vi "Main Window.vi"() -> ()   [LabVIEW 2015]
uses:
  Control Button/Exit.ctl
  Control Button/login.ctl
  Control Button/Logout.ctl
  Control Button/setting.ctl
  Control Button/report.ctl
  Control Button/Manual.ctl
  Control Button/Start.ctl
  Enqueue/Main window Seq/Test selection_1.ctl
  Enqueue/Main window Seq/Test seq_1.ctl
  Galobal variable_TI.vi
  Project Setup/Globle Variable/GR_Servo.vi
panel:
  out "Boolean 3":bool
  out "error out 2":errorcluster
  out "Boolean 2":bool
  out "Error 2":bool
  out "Error":bool
  out "User Name":string
  out "error out":errorcluster
  out "x = y?":bool
  out "Company Name":string
  in  "Sign In":T1
  out "Boolean":bool
  in  "Dashbord":T6
  in  "Login Window":T8 {"User Name" items=["admin", "mmum", "a", "AJAY Kumar", "", "", "", "", "", "", "", "", "", "", "", "", "", "", "", "", "", "", "", "", "", "", "", "", "", "", "", ""]}
  in  "Exit":T9
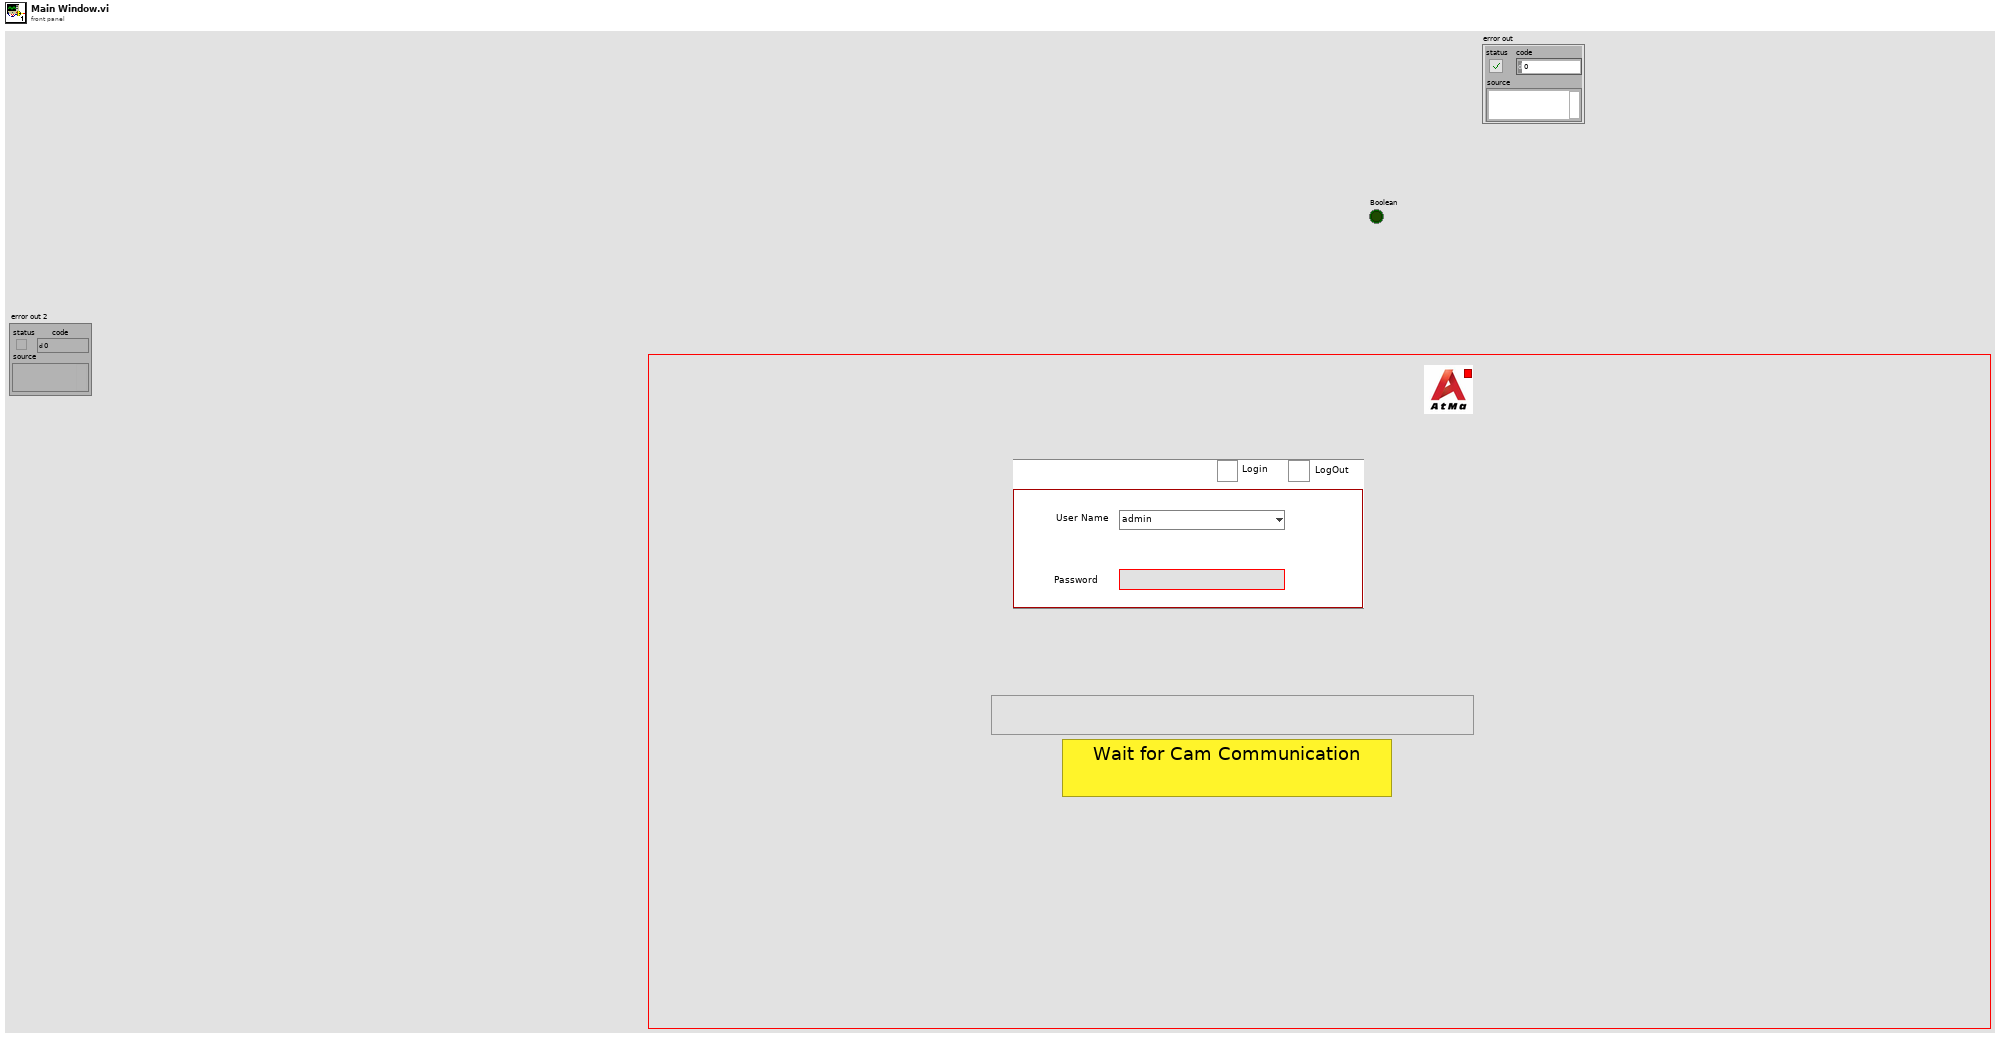
[diagram p1: front panel]
types:
  T1 = typedef "login.ctl" = bool
  T2 = typedef "setting.ctl" = bool
  T3 = typedef "report.ctl" = bool
  T4 = typedef "Manual.ctl" = bool
  T5 = typedef "Start.ctl" = bool
  T6 = cluster{"Setting":T2, "Report":T3, "Manaul":T4, "Start":T5}
  T7 = typedef "Logout.ctl" = bool
  T8 = cluster{"User Name":u16, "Password":string, "Sign In":T1, "Log Out":T7}
  T9 = typedef "Exit.ctl" = bool
  T10 = typedef "Test selection_1.ctl" = enum16{"Init", "Enqueue ", "Enqueue N", "Enqueue in stack", "Enqueue in stack N", "Dequeue", "Dequeue N", "Flush", "Release Queue"}
  T11 = typedef "Test seq_1.ctl" = enum16{"Poll Event", "Login", "Logout", "Confi", "Manual", "Report", "Testing", "Exit"}
  T12 = cluster{"XInput":dbl[], "Y New Value":dbl[], "Avg point":i16}[]
  T13 = cluster{"Slop":dbl[], "Intercept":dbl[], "Average ":i16[]}
  T14 = cluster{"UserName":string[], "Password":string[], "Usertype":string[], "Analog Min":string[], "Analog Max":string[], "DigitalInput Port":string[], "Digital Output Port":string[], "ANalog Port":string[], "IOList":cluster{"DI List_280":string[], "D0List _280":string[], "AI List_280":string[]}}
  T15 = cluster{"DI List_280":string[], "D0List _280":string[], "AI List_280":string[]}
  T16 = cluster{"DigitalInput Port[0]":string, "DigitalInput Port[1]":string, "DigitalInput Port[2]":string, "DigitalInput Port[3]":string, "DigitalInput Port[4]":string, "DigitalInput Port[5]":string, "DigitalInput Port[6]":string, "DigitalInput Port[7]":string, "DigitalInput Port[8]":string, "DigitalInput Port[9]":string, "DigitalInput Port[10]":string, "DigitalInput Port[11]":string, "DigitalInput Port[12]":string, "DigitalInput Port[13]":string, "DigitalInput Port[14]":string, "DigitalInput Port[15]":string}
  T17 = cluster{"Digital Output Port[0]":string, "Digital Output Port[1]":string, "Digital Output Port[2]":string, "Digital Output Port[3]":string, "Digital Output Port[4]":string, "Digital Output Port[5]":string, "Digital Output Port[6]":string, "Digital Output Port[7]":string, "Digital Output Port[8]":string, "Digital Output Port[9]":string, "Digital Output Port[10]":string, "Digital Output Port[11]":string, "Digital Output Port[12]":string, "Digital Output Port[13]":string, "Digital Output Port[14]":string, "Digital Output Port[15]":string, "Digital Output Port[16]":string, "Digital Output Port[17]":string, "Digital Output Port[18]":string, "Digital Output Port[19]":string, "Digital Output Port[20]":string, "Digital Output Port[21]":string, "Digital Output Port[22]":string, "Digital Output Port[23]":string, "Digital Output Port[24]":string, "Digital Output Port[25]":string, "Digital Output Port[26]":string, "Digital Output Port[27]":string, "Digital Output Port[28]":string, "Digital Output Port[29]":string}
  T18 = cluster{"ANalog Port[0]":string, "ANalog Port[1]":string, "ANalog Port[2]":string, "ANalog Port[3]":string, "ANalog Port[4]":string, "ANalog Port[5]":string, "ANalog Port[6]":string, "ANalog Port[7]":string, "ANalog Port[8]":string, "ANalog Port[9]":string, "ANalog Port[10]":string, "ANalog Port[11]":string, "ANalog Port[12]":string, "ANalog Port[13]":string, "ANalog Port[14]":string, "ANalog Port[15]":string, "ANalog Port[16]":string, "ANalog Port[17]":string, "ANalog Port[18]":string, "ANalog Port[19]":string, "ANalog Port[20]":string, "ANalog Port[21]":string, "ANalog Port[22]":string, "ANalog Port[23]":string, "ANalog Port[24]":string, "ANalog Port[25]":string, "ANalog Port[26]":string, "ANalog Port[27]":string, "ANalog Port[28]":string, "ANalog Port[29]":string, "ANalog Port[30]":string, "ANalog Port[31]":string}
  T19 = enum32{"Invalid", "Standard", "Closed", "Hidden", "Minimized", "Maximized"}
  T20 = enum8{"Enabled", "Disabled", "Disabled and Grayed Out"}
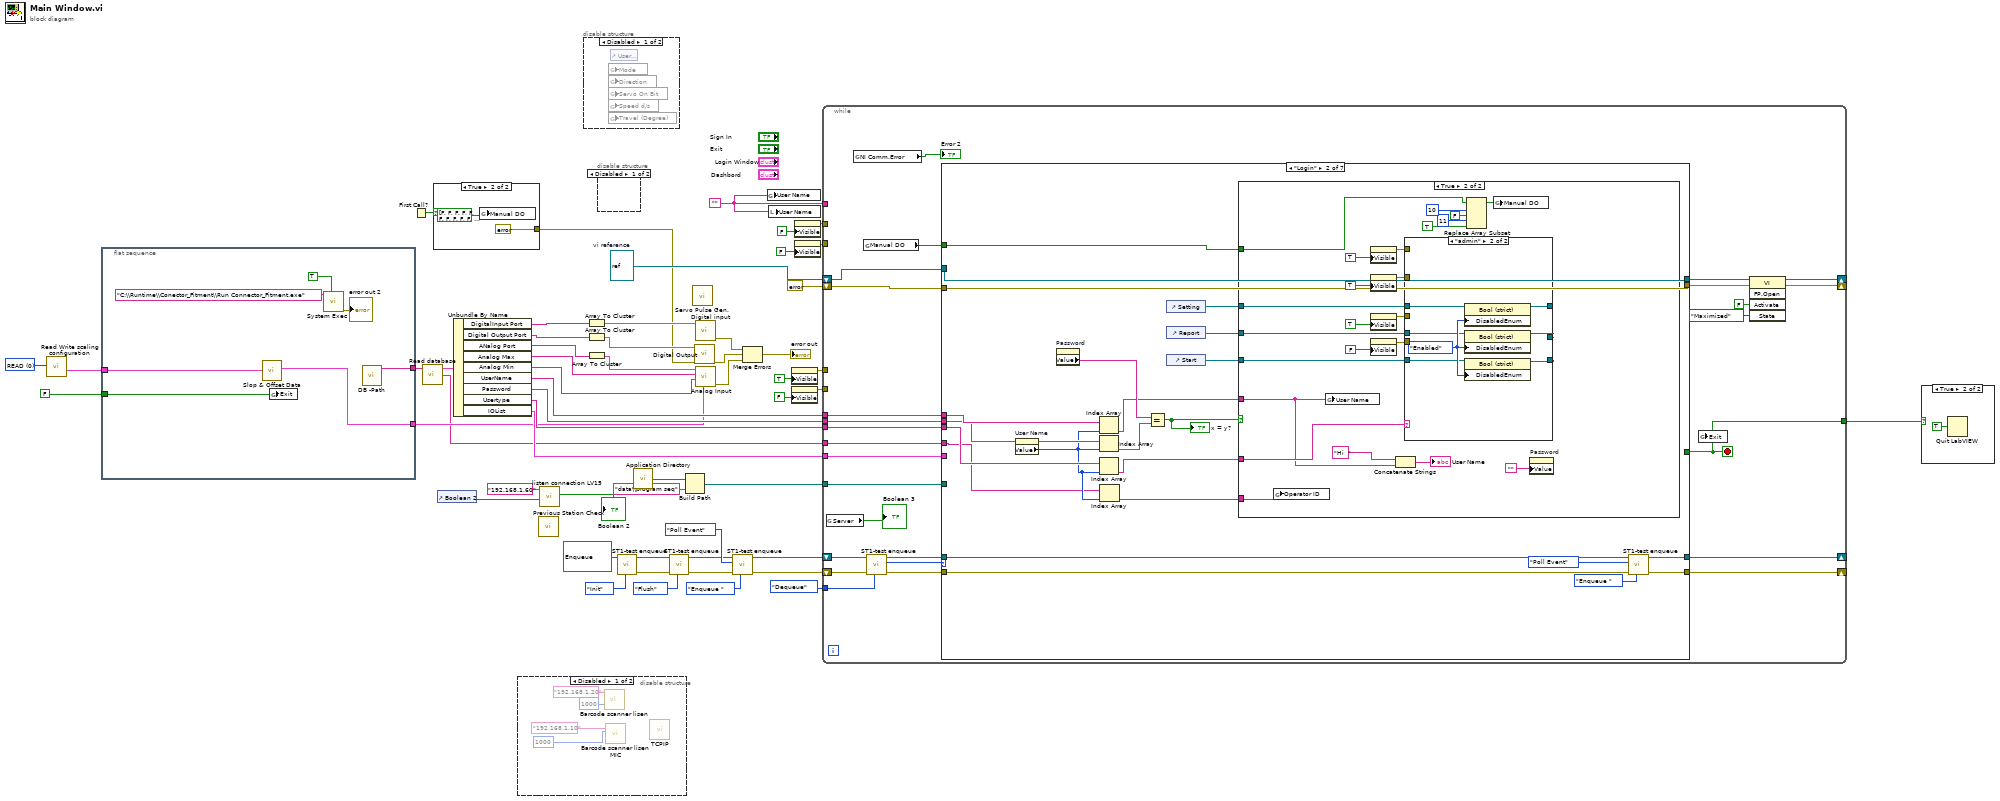
[diagram p0: block diagram]
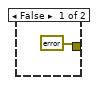
[diagram p5: hidden frame]
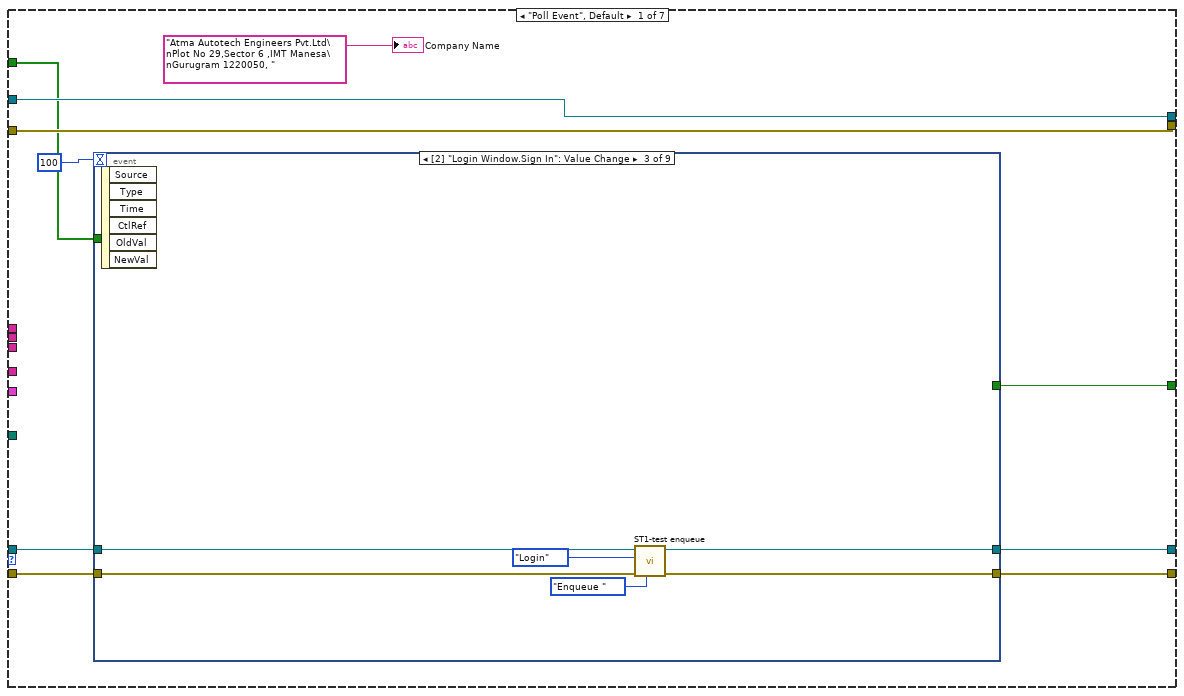
[diagram p7: hidden frame]
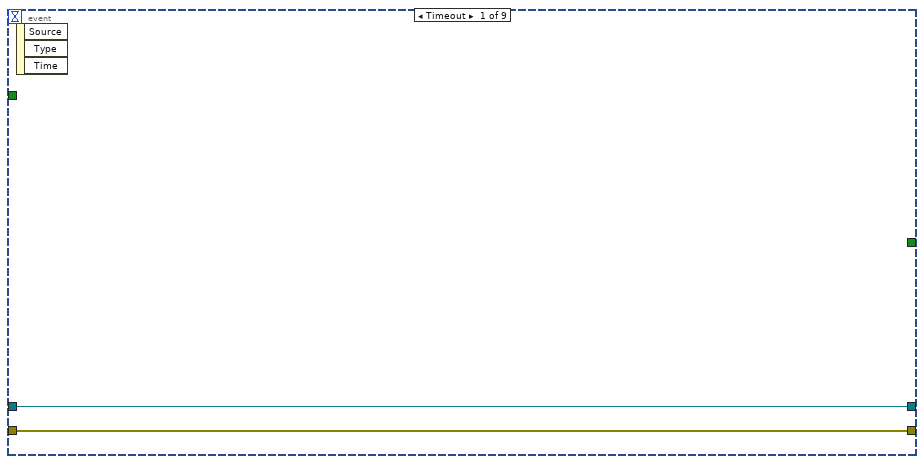
[diagram p8: hidden frame]
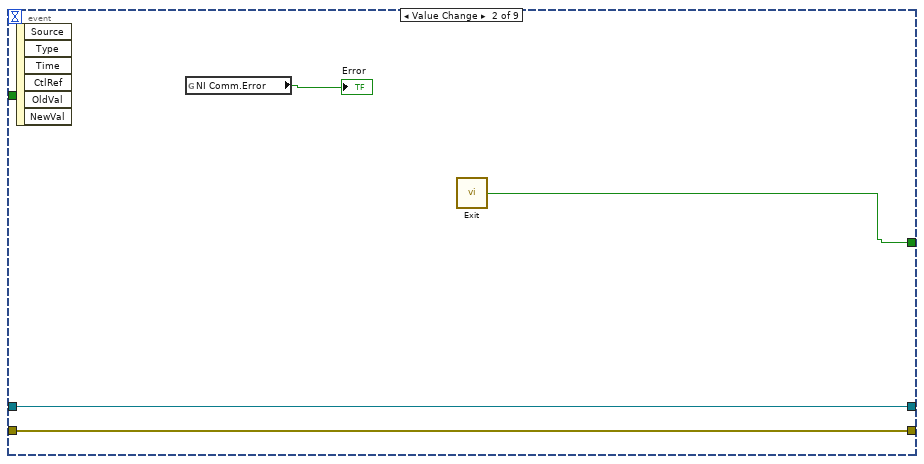
[diagram p9: hidden frame]
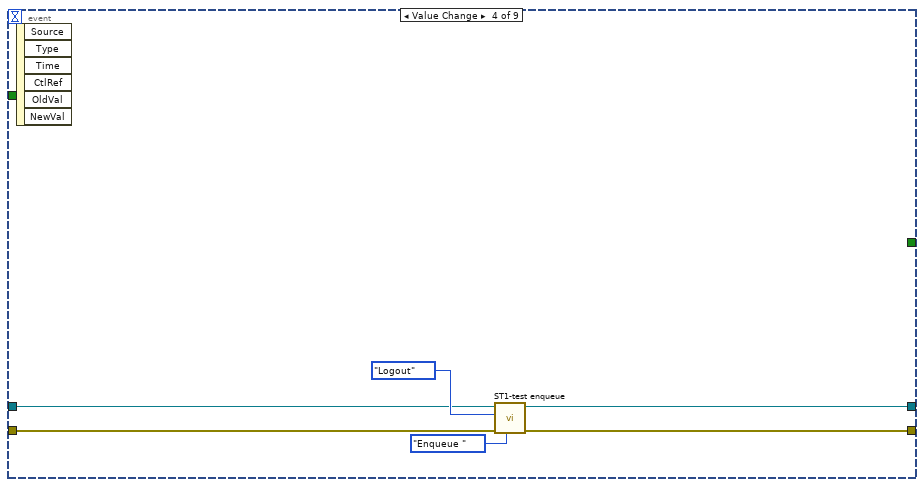
[diagram p10: hidden frame]
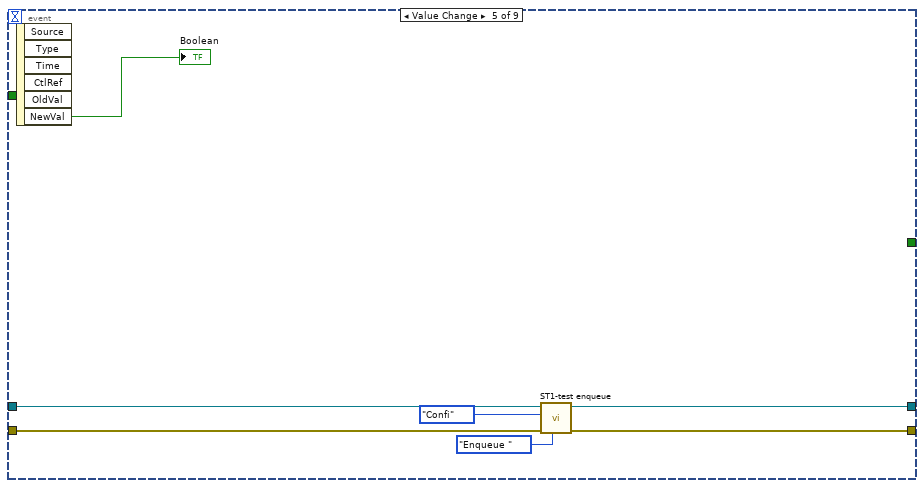
[diagram p11: hidden frame]
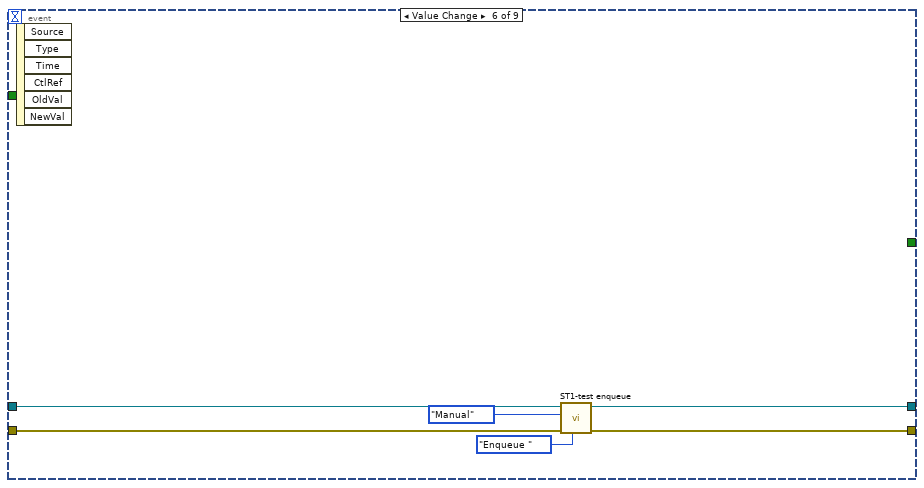
[diagram p12: hidden frame]
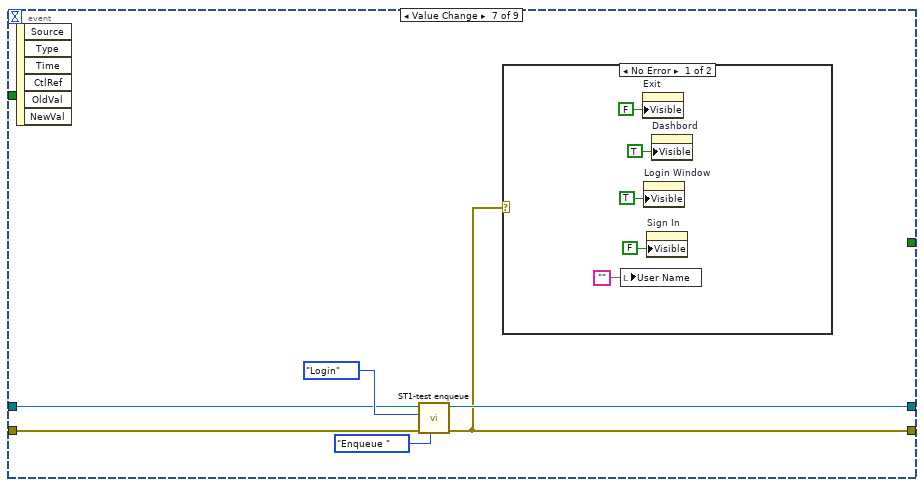
[diagram p13: hidden frame]
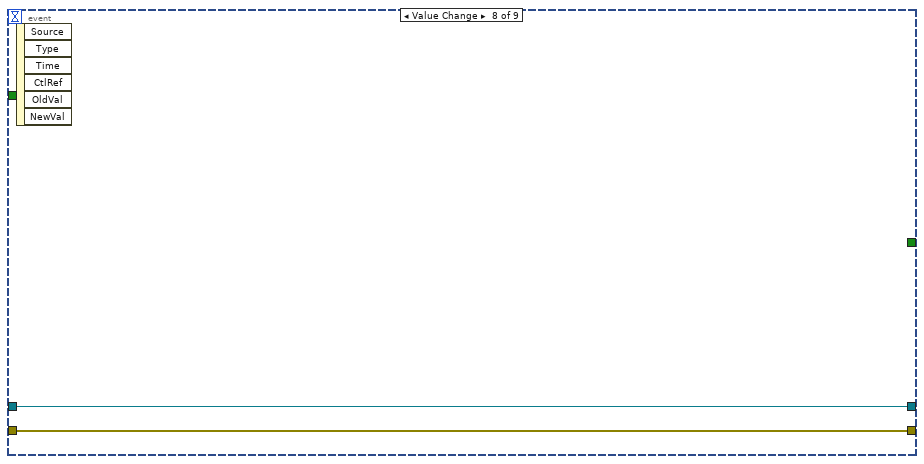
[diagram p15: hidden frame]
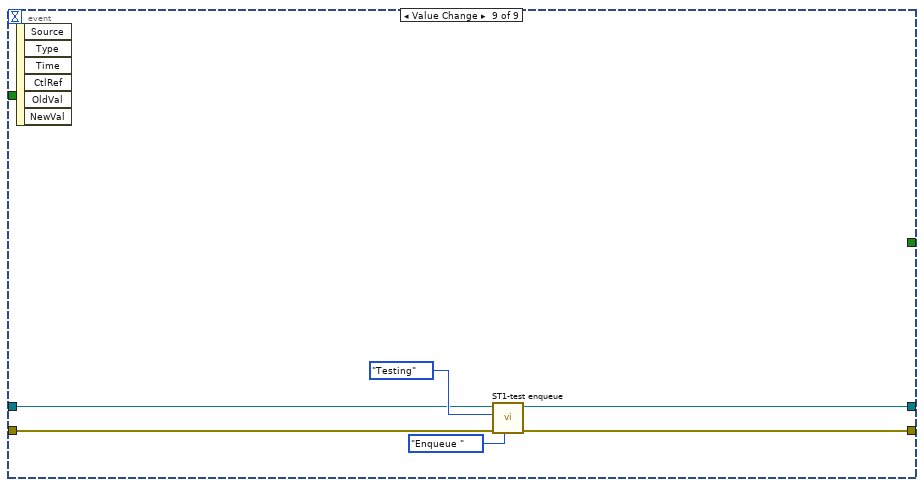
[diagram p16: hidden frame]
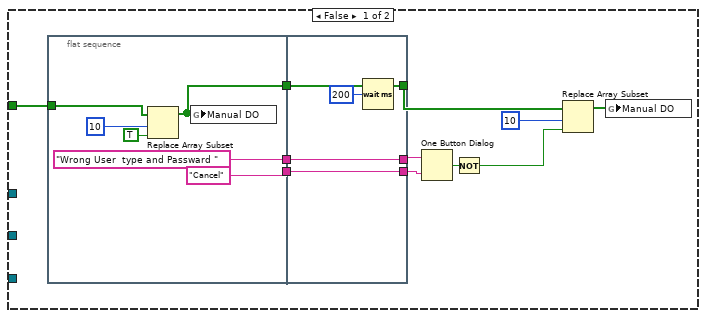
[diagram p17: hidden frame]
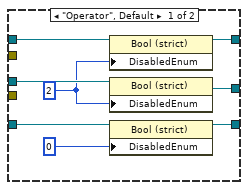
[diagram p18: hidden frame]
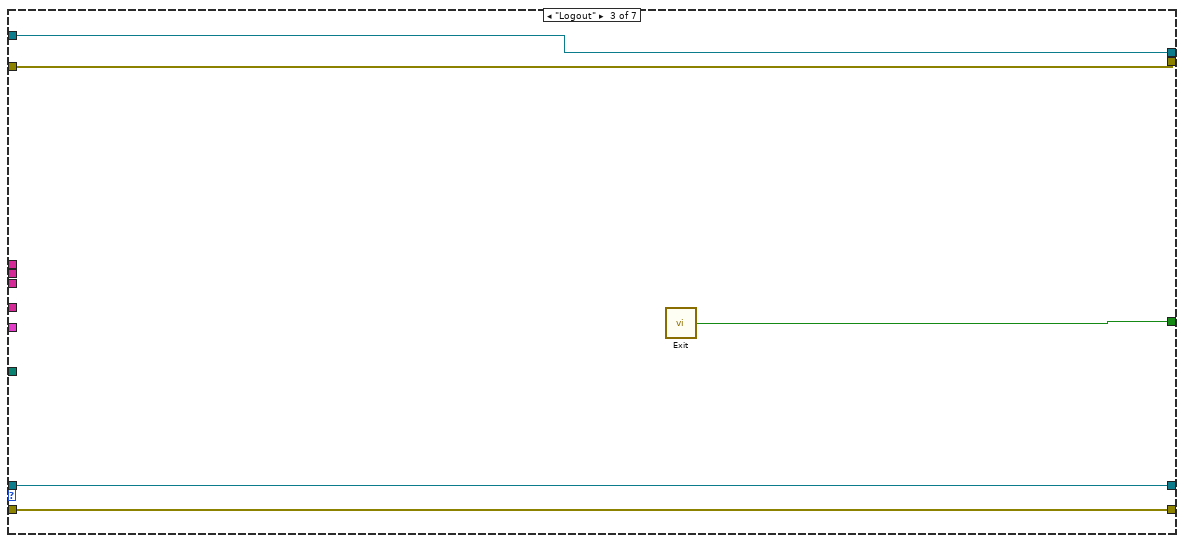
[diagram p19: hidden frame]
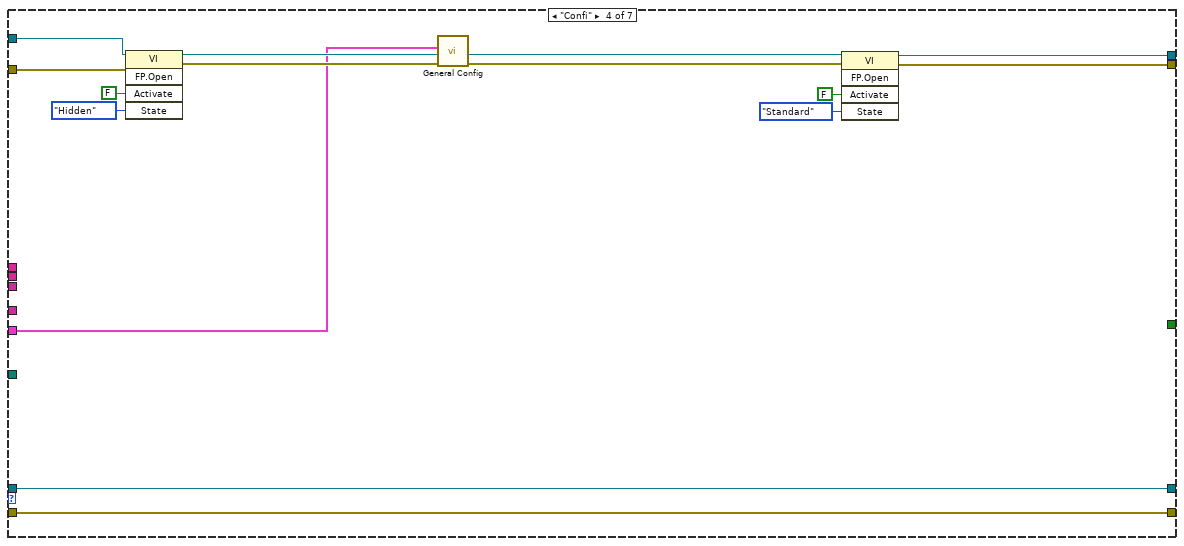
[diagram p20: hidden frame]
diagram:
  w18 = u16 0 items=["READ", "WRITE"] ("Read/Write")
  w33 = ""
  w43 = refnum<vi> refnum  # vi reference
  w44 = refnum<queue> refnum items=["Poll Event", "Login", "Logout", "Confi", "Manual", "Report", "Testing", "Exit"] ("queue in")
  n1 = call "Read Write scaling configuration.vi"("Read/Write"=w18) -> ("Output"=w17:T12)  [unwired: 4 in, 2 out]
  n2 = flat-sequence {
    tunnel: [w62] -> w32
    tunnel: w17 -> [w61]
    tunnel: [w60] -> w16
    tunnel: FALSE ("Exit") -> [w59]
    frame #0 {
      n3 = call "Slop & Offset Data.vi"("Input"=w61) -> ("Cluster"=w60:T13)  [unwired: 10 in]
      n4 = global write "Galobal variable_TI.vi" "Exit"(w59) -> ()
      n5 = call <vilib>:"System Exec.vi"("wait until completion? (T)"=TRUE, "command line"="C:\\Runtime\\Conector_Fitment\\Run Connector_Fitment.exe") -> ("error out"=→"error out 2":errorcluster)  [unwired: 6 in, 3 out]
      n6 = call "DB -Path.vi"() -> ("String"=w62:string)  [unwired: 11 in]
    }
  }
  n7 = First Call?() -> (First Call?: T/F=w7:bool)
  n8 = call "Read database.vi"("String"=w32) -> ("Operator Id"=w1:string[], "DB Data"=w31:T14)  [unwired: 2 in, 1 out]
  n9 = case shown="True" w7 {
    tunnel: [errorcluster {"status"=FALSE, "code"=0, "source"=""} ("error constant") errorcluster {"status"=FALSE, "code"=0, "source"=""} ("error constant")] -> w6
    frame False {
    }
    frame True {
      n10 = global write "Galobal variable_TI.vi" "Manual DO"(bool[] [FALSE, FALSE, FALSE, FALSE, FALSE, FALSE, FALSE, FALSE, FALSE, FALSE, FALSE, FALSE, FALSE, FALSE, FALSE, FALSE, FALSE, FALSE, FALSE, FALSE, FALSE, FALSE, FALSE, FALSE, FALSE, FALSE, FALSE, FALSE, FALSE, FALSE] ("Manual DO")) -> ()
    }
  }
  n11 = control-ref of="Boolean 2"() -> (w3:refnum<vi>)
  n12 = Unbundle By Name(w31) -> ("DigitalInput Port"=w30:string[], "Digital Output Port"=w28:string[], "ANalog Port"=w26:string[], "Analog Max"=w24:string[], "Analog Min"=w23:string[], "UserName"=w22:string[], "Password"=w21:string[], "Usertype"=w20:string[], "IOList"=w19:T15)
  n13 = disable-structure shown="Disabled" {
    frame Disabled {
      n14 = call "Barcode scanner lisen.vi"("port"=u16 1000, "service name"="192.168.1.20") -> ()  [unwired: 7 in, 3 out]
      n15 = call "Barcode scanner lisen MIC.vi"("port"=u16 1000, "service name"="192.168.1.10") -> ()  [unwired: 7 in, 3 out]
      n16 = call "TCPIP.vi"() -> ()  [unwired: 12 in]
    }
    frame Enabled {
    }
  }
  n17 = call "Previous Station Check.vi"() -> ()  [unwired: 12 in]
  n18 = call "listen connection LV15.vi"("Bool Refnum"=w3, "service name"="192.168.1.60") -> ("Boolean 3"=→"Boolean 2":bool)  [unwired: 7 in, 1 out]
  n19 = disable-structure shown="Disabled" {
    frame Disabled {
      n20 = global read "GR_Servo.vi" "Mode"() -> ()  [unwired: 1 in]
      n21 = global read "GR_Servo.vi" "Direction"() -> ()  [unwired: 1 in]
      n22 = global read "GR_Servo.vi" "Servo On Bit"() -> ()  [unwired: 1 in]
      n23 = global read "GR_Servo.vi" "Speed d/s"() -> ()  [unwired: 1 in]
      n24 = global read "GR_Servo.vi" "Travel (Degree)"() -> ()  [unwired: 1 in]
      n25 = control-ref of="User Name"() -> ()  [unwired: 1 out]
    }
    frame Enabled {
    }
  }
  n26 = Array To Cluster(array=w30) -> (cluster=w29:T16)
  n27 = Array To Cluster(array=w28) -> (cluster=w27:T17)
  n28 = Array To Cluster(array=w26) -> (cluster=w25:T18)
  n29 = disable-structure shown="Disabled" {
    frame Disabled {
    }
    frame Enabled {
    }
  }
  n30 = call "ST1-test enqueue.vi"("Enum Selection"=Test_selection_1."Init", "queue in"=w44) -> ("error out"=w53:errorcluster, "queue Out"=w49:refnum<queue>)  [unwired: 6 in, 1 out]
  n31 = call <vilib>:"Application Directory.vi"() -> ("Application Directory"=w10:path)
  n32 = call "ST1-test enqueue.vi"("Enum Selection"=Test_selection_1."Flush", "Error In"=w53, "queue in"=w49) -> ("error out"=w51:errorcluster, "queue Out"=w48:refnum<queue>)  [unwired: 5 in, 1 out]
  n33 = Build Path(base path=w10, name or relative path="data\\program seq") -> (appended path=w8:path)
  n34 = call "Servo Pulse Gen..vi"() -> ()  [unwired: 12 in]
  n35 = call "Digital Output.vi"("error in"=w6, "DAQmx OutPut Setting"=w27) -> ("error out"=w14:errorcluster)  [unwired: 8 in, 1 out]
  n36 = call "Digital input.vi"("DAQmx InPut Setting"=w29) -> ("error out"=w12:errorcluster)  [unwired: 9 in, 1 out]
  n37 = call "Analog Input.vi"("clai. Parmeter"=w16, "Min Value"=w23, "Max Value"=w24, "DAQmx Analog Input Setting"=w25) -> ("error out"=w13:errorcluster)  [unwired: 6 in, 1 out]
  n38 = call "ST1-test enqueue.vi"("Enum Selection"=Test_selection_1."Enqueue ", "Error In"=w51, "Enqueue"=Test_seq_1."Poll Event", "queue in"=w48) -> ("error out"=w46:errorcluster, "queue Out"=w47:refnum<queue>)  [unwired: 4 in, 1 out]
  n39 = Merge Errors(w12, w14, w13) -> (→"error out":errorcluster)
  n40 = global write "Galobal variable_TI.vi" "User Name"(w33) -> ()
  n41 = local write "User Name"(w33) -> ()
  n42 = property on="Login Window" class="Clust (strict)"("Visible"=TRUE) -> (error out=w38:errorcluster)  [unwired: 2 in, 1 out]
  n43 = property on="Sign In" class="Bool (strict)"("Visible"=FALSE) -> (error out=w37:errorcluster)  [unwired: 2 in, 1 out]
  n44 = property on="Exit" class="Bool (strict)"("Visible"=FALSE) -> (error out=w35:errorcluster)  [unwired: 2 in, 1 out]
  n45 = property on="Dashbord" class="Clust (strict)"("Visible"=FALSE) -> (error out=w40:errorcluster)  [unwired: 2 in, 1 out]
  n46 = while {
    shift-right: [w89] -> _
    shift-left: w47 -> [w95]
    shift-right: [w88] -> _
    shift-left: w46 -> [w94]
    tunnel: Test_selection_1."Dequeue" ("Enum Selection") -> [w93]
    shift-right: [w80] -> _
    shift-left: errorcluster {"status"=FALSE, "code"=0, "source"=""} ("error out") -> [w86]
    shift-right: [w81] -> _
    shift-left: w43 -> [w87]
    tunnel: w40 -> [_]
    tunnel: w38 -> [_]
    tunnel: w37 -> [_]
    tunnel: w35 -> [_]
    tunnel: w33 -> [_]
    tunnel: w22 -> [w79]
    tunnel: w21 -> [w78]
    tunnel: w20 -> [w77]
    tunnel: w19 -> [w76]
    tunnel: w8 -> [w75]
    tunnel: [w73] -> w5
    tunnel: w1 -> [w70]
    stop <- w73 stop-if-true
    n47 = global read "Galobal variable_TI.vi" "Server"() -> (→"Boolean 3":bool)
    n48 = global read "Galobal variable_TI.vi" "NI Comm.Error"() -> (→"Error 2":bool)
    n49 = global read "Galobal variable_TI.vi" "Manual DO"() -> (w74:bool[])
    n50 = call "ST1-test enqueue.vi"("Enum Selection"=w93, "Error In"=w94, "queue in"=w95) -> ("error out"=w90:errorcluster, "D-enqueue"=w92:T11, "queue Out"=w91:refnum<queue>)  [unwired: 5 in]
    n51 = case shown="\"Login\"" w92 {
      tunnel: [w103 _ w238 _ _ _ _] -> w73
      tunnel: w91 -> [w104 w160 w242 w256 w264 w273 w290]
      tunnel: w90 -> [w105 w159 w241 w255 w263 w272 w289]
      tunnel: [w102 w163 w242 w256 w264 w273 w290] -> w89
      tunnel: [w101 w162 w241 w255 w263 w272 w289] -> w88
      tunnel: [w100 w172 w240 w250 w259 w271 w276] -> w83
      tunnel: [w99 w171 w239 w249 w260 w270 w274] -> w82
      tunnel: w87 -> [w100 w172 w240 w248 w261 w271 w282]
      tunnel: w86 -> [w99 w171 w239 w247 w262 w270 w285]
      tunnel: w79 -> [_ w169 _ _ _ _ _]
      tunnel: w78 -> [_ w168 _ _ _ _ _]
      tunnel: w77 -> [_ w167 _ _ _ _ _]
      tunnel: w76 -> [_ _ _ w243 w258 _ w288]
      tunnel: w75 -> [_ _ _ _ _ _ w280]
      tunnel: w74 -> [w96 w161 _ _ _ _ _]
      tunnel: w70 -> [_ w157 _ _ _ _ _]
      frame "Poll Event", Default {
        n52 = event shown="[2] \"Login Window.Sign In\": Value Change" {
          selector: _ -> [_ _ _ _ _ _ _ _ _]
          dyn-events: _ -> [_ _ _ _ _ _ _ _ _]
          timeout: 100 -> [_ _ _ _ _ _ _ _ _]
          tunnel: [_ w109 _ _ _ _ _ _ _] -> w103
          tunnel: w105 -> [w106 w110 w115 w118 w126 w134 w140 w148 w152]
          tunnel: w104 -> [w107 w111 w116 w119 w127 w132 w139 w149 w153]
          tunnel: [w107 w111 w114 w121 w125 w131 w138 w149 w151] -> w102
          tunnel: [w106 w110 w113 w120 w124 w133 w137 w148 w150] -> w101
          tunnel: w96 -> [_ _ _ _ _ _ _ _ _]
          event Timeout {
            n53 = event-data() -> ()  [unwired: 1 in, 3 out]
          }
          event Value Change {
            n54 = event-data() -> ()  [unwired: 1 in, 6 out]
            n55 = global read "Galobal variable_TI.vi" "NI Comm.Error"() -> (→"Error":bool)
            n56 = call "Exit.vi"() -> ("Exit"=w109:bool)  [unwired: 1 in]
          }
          event Value Change {
            n57 = event-data() -> ()  [unwired: 1 in, 6 out]
            n58 = call "ST1-test enqueue.vi"("Enum Selection"=Test_selection_1."Enqueue ", "Error In"=w115, "Enqueue"=Test_seq_1."Login", "queue in"=w116) -> ("error out"=w113:errorcluster, "queue Out"=w114:refnum<queue>)  [unwired: 4 in, 1 out]
          }
          event Value Change {
            n59 = event-data() -> ()  [unwired: 1 in, 6 out]
            n60 = call "ST1-test enqueue.vi"("Enum Selection"=Test_selection_1."Enqueue ", "Error In"=w118, "Enqueue"=Test_seq_1."Logout", "queue in"=w119) -> ("error out"=w120:errorcluster, "queue Out"=w121:refnum<queue>)  [unwired: 4 in, 1 out]
          }
          event Value Change {
            n61 = event-data() -> ("NewVal"=→"Boolean":T2)  [unwired: 1 in, 5 out]
            n62 = call "ST1-test enqueue.vi"("Enum Selection"=Test_selection_1."Enqueue ", "Error In"=w126, "Enqueue"=Test_seq_1."Confi", "queue in"=w127) -> ("error out"=w124:errorcluster, "queue Out"=w125:refnum<queue>)  [unwired: 4 in, 1 out]
          }
          event Value Change {
            n63 = event-data() -> ()  [unwired: 1 in, 6 out]
            n64 = call "ST1-test enqueue.vi"("Enum Selection"=Test_selection_1."Enqueue ", "Error In"=w134, "Enqueue"=Test_seq_1."Manual", "queue in"=w132) -> ("error out"=w133:errorcluster, "queue Out"=w131:refnum<queue>)  [unwired: 4 in, 1 out]
          }
          event Value Change {
            n65 = event-data() -> ()  [unwired: 1 in, 6 out]
            n66 = call "ST1-test enqueue.vi"("Enum Selection"=Test_selection_1."Enqueue ", "Error In"=w140, "Enqueue"=Test_seq_1."Login", "queue in"=w139) -> ("error out"=w137:errorcluster, "queue Out"=w138:refnum<queue>)  [unwired: 4 in, 1 out]
            n67 = case shown="No Error" w137 {
              frame No Error {
                n68 = local write "User Name"("") -> ()
                n69 = property on="Exit" class="Bool (strict)"("Visible"=FALSE) -> ()  [unwired: 2 in, 2 out]
                n70 = property on="Login Window" class="Clust (strict)"("Visible"=TRUE) -> ()  [unwired: 2 in, 2 out]
                n71 = property on="Sign In" class="Bool (strict)"("Visible"=FALSE) -> ()  [unwired: 2 in, 2 out]
                n72 = property on="Dashbord" class="Clust (strict)"("Visible"=TRUE) -> ()  [unwired: 2 in, 2 out]
              }
              frame Error {
              }
            }
          }
          event Value Change {
            n73 = event-data() -> ()  [unwired: 1 in, 6 out]
          }
          event Value Change {
            n74 = event-data() -> ()  [unwired: 1 in, 6 out]
            n75 = call "ST1-test enqueue.vi"("Enum Selection"=Test_selection_1."Enqueue ", "Error In"=w152, "Enqueue"=Test_seq_1."Testing", "queue in"=w153) -> ("error out"=w150:errorcluster, "queue Out"=w151:refnum<queue>)  [unwired: 4 in, 1 out]
          }
        }
        "Company Name" <- "Atma Autotech Engineers Pvt.Ltd\nPlot No 29,Sector 6 ,IMT Manesa\nGurugram 1220050, " ("string")
      }
      frame "Login" {
        n76 = property on="User Name" class="Ring (strict)"() -> ("Value"=w158:u16)  [unwired: 2 in, 2 out]
        n77 = property on="Password" class="Str"() -> ("Value"=w177:string)  [unwired: 2 in, 2 out]
        n78 = Index Array(array=w169, index=w158) -> (element=w170:string)
        n79 = Index Array(array=w168, index=w158) -> (element=w178:string)
        n80 = Index Array(array=w167, index=w158) -> (element=w176:string)
        n81 = Index Array(array=w157, index=w158) -> (element=w156:string)
        n82 = Equal?(x=w177, y=w178) -> (x = y?=w166:bool)
        "x = y?" <- w166
        n83 = control-ref of="Setting"() -> (w175:refnum<vi>)
        n84 = control-ref of="Report"() -> (w173:refnum<vi>)
        n85 = control-ref of="Start"() -> (w174:refnum<vi>)
        n86 = case shown="True" w166 {
          tunnel: w176 -> [_ w218]
          tunnel: w175 -> [_ w222]
          tunnel: w173 -> [_ w221]
          tunnel: w174 -> [_ w220]
          tunnel: w170 -> [_ w201]
          tunnel: w161 -> [w189 w205]
          tunnel: w156 -> [_ w200]
          frame False {
            n87 = flat-sequence {
              tunnel: w189 -> [w195]
              tunnel: ["Wrong User  type and Passward " ("message")] -> w186
              tunnel: ["Cancel" ("button name (\"OK\")")] -> w185
              tunnel: [w190] -> w182
              tunnel: [w198] -> w187
              tunnel: [w199] -> w188
              tunnel: w186 -> [w199]
              tunnel: w185 -> [w198]
              tunnel: [w196] -> w181
              tunnel: w182 -> [w196]
              frame #0 {
                n88 = Replace Array Subset(array=w195, new element=TRUE ("new element/subarray"), index=10) -> (w190:bool[])
                n89 = global write "Galobal variable_TI.vi" "Manual DO"(w190) -> ()
              }
              frame #1 {
                n90 = Wait (ms)(milliseconds to wait=u32 200) -> ()  [unwired: 1 out]
              }
            }
            n91 = One Button Dialog(message=w188, button name ("OK")=w187) -> (true=w180:bool)
            n92 = Not(x=w180) -> (.not. x?=w179:bool)
            n93 = Replace Array Subset(array=w181, new element=w179, index=10) -> (w184:bool[])
            n94 = global write "Galobal variable_TI.vi" "Manual DO"(w184) -> ()
          }
          frame True {
            n95 = global write "Galobal variable_TI.vi" "Operator ID"(w200) -> ()
            n96 = global write "Galobal variable_TI.vi" "User Name"(w201) -> ()
            n97 = property on="Exit" class="Bool (strict)"("Visible"=TRUE) -> (error out=w209:errorcluster)  [unwired: 2 in, 1 out]
            n98 = property on="Dashbord" class="Clust (strict)"("Visible"=TRUE) -> (error out=w214:errorcluster)  [unwired: 2 in, 1 out]
            n99 = property on="Sign In" class="Bool (strict)"("Visible"=TRUE) -> (error out=w213:errorcluster)  [unwired: 2 in, 1 out]
            n100 = property on="Login Window" class="Clust (strict)"("Visible"=FALSE) -> (error out=w215:errorcluster)  [unwired: 2 in, 1 out]
            n101 = Concatenate Strings("Hi  " ("string"), w201) -> (→"User Name":string)
            n102 = case shown="\"admin\"" w218 {
              tunnel: [w230 w236] -> _
              tunnel: [w229 w235] -> _
              tunnel: [w228 w234] -> _
              tunnel: w222 -> [w227 w233]
              tunnel: w221 -> [w226 w232]
              tunnel: w220 -> [w225 w231]
              tunnel: w215 -> [_ _]
              tunnel: w214 -> [_ _]
              tunnel: w213 -> [_ _]
              tunnel: w209 -> [_ _]
              frame "Operator", Default {
                w223 = 2
                n103 = property class="Bool (strict)"(reference=w227, "DisabledEnum"=w223) -> (reference out=w230:refnum<vi>)  [unwired: 1 in, 1 out]
                n104 = property class="Bool (strict)"(reference=w226, "DisabledEnum"=w223) -> (reference out=w229:refnum<vi>)  [unwired: 1 in, 1 out]
                n105 = property class="Bool (strict)"(reference=w225, "DisabledEnum"=0) -> (reference out=w228:refnum<vi>)  [unwired: 1 in, 1 out]
              }
              frame "admin" {
                w237 = T20."Enabled" ("Disabled")
                n106 = property class="Bool (strict)"(reference=w233, "DisabledEnum"=w237) -> (reference out=w236:refnum<vi>)  [unwired: 1 in, 1 out]
                n107 = property class="Bool (strict)"(reference=w232, "DisabledEnum"=w237) -> (reference out=w235:refnum<vi>)  [unwired: 1 in, 1 out]
                n108 = property class="Bool (strict)"(reference=w231, "DisabledEnum"=w237) -> (reference out=w234:refnum<vi>)  [unwired: 1 in, 1 out]
              }
            }
            n109 = Replace Array Subset(array=w205, new element #1=FALSE ("new element/subarray"), index #1=10 ("index"), new element #2=TRUE ("new element/subarray"), index #2=11 ("index")) -> (w206:bool[])
            n110 = global write "Galobal variable_TI.vi" "Manual DO"(w206) -> ()
            n111 = property on="Password" class="Str"("Value"="") -> ()  [unwired: 2 in, 2 out]
          }
        }
        n112 = call "ST1-test enqueue.vi"("Enum Selection"=Test_selection_1."Enqueue ", "Error In"=w159, "Enqueue"=Test_seq_1."Poll Event", "queue in"=w160) -> ("error out"=w162:errorcluster, "queue Out"=w163:refnum<queue>)  [unwired: 4 in, 1 out]
      }
      frame "Logout" {
        n113 = call "Exit.vi"() -> ("Exit"=w238:bool)  [unwired: 1 in]
      }
      frame "Confi" {
        n114 = invoke class="VI" method="FP.Open"(reference=w248, error in=w247, "Activate"=FALSE ("Activate?"), "State"=T19."Hidden") -> (reference out=w244:refnum<vi>, error out=w246:errorcluster)  [unwired: 1 in, 3 out]
        n115 = call "General Config.vi"("error In"=w246, "IOList"=w243) -> ("error out"=w245:errorcluster)  [unwired: 8 in, 1 out]
        n116 = invoke class="VI" method="FP.Open"(reference=w244, error in=w245, "Activate"=FALSE ("Activate?"), "State"=T19."Standard") -> (reference out=w250:refnum<vi>, error out=w249:errorcluster)  [unwired: 1 in, 3 out]
      }
      frame "Manual" {
        w257 = TRUE ("Manual CMD")
        n117 = global write "Galobal variable_TI.vi" "Manual CMD"(w257) -> ()
        n118 = flat-sequence {
          tunnel: w262 -> [w269]
          tunnel: w261 -> [w268]
          tunnel: [w267] -> w260
          tunnel: [w266] -> w259
          tunnel: w258 -> [w265]
          tunnel: w257 -> [_]
          frame #0 {
            n119 = call "Manual.vi"("vi reference"=w268, "error in (no error)"=w269, "IOList_280"=w265) -> ("error out"=w267:errorcluster, "Out reference"=w266:refnum<vi>)  [unwired: 7 in]
          }
        }
      }
      frame "Report" {
      }
      frame "Testing" {
        n120 = Unbundle By Name(w288) -> ("DI List_280"=w281:string[])
        n121 = invoke class="VI" method="FP.Open"(reference=w282, error in=w285, "Activate"=FALSE ("Activate?"), "State"=T19."Hidden") -> (reference out=w284:refnum<vi>, error out=w283:errorcluster)  [unwired: 1 in, 3 out]
        n122 = call "Program list Selection.vi"("error in"=w283, "FeedBack Channel"=w281, "Filepath"=w280, "vi referenceIn"=w284) -> ("error out"=w275:errorcluster, "vi reference Out"=w277:refnum<vi>)  [unwired: 4 in, 2 out]
        n123 = invoke class="VI" method="FP.Open"(reference=w277, error in=w275, "Activate"=FALSE ("Activate?"), "State"=T19."Standard") -> (reference out=w276:refnum<vi>, error out=w274:errorcluster)  [unwired: 1 in, 3 out]
      }
    }
    n124 = global write "Galobal variable_TI.vi" "Exit"(w73) -> ()
    n125 = invoke class="VI" method="FP.Open"(reference=w83, error in=w82, "Activate"=FALSE ("Activate?"), "State"=T19."Maximized") -> (reference out=w81:refnum<vi>, error out=w80:errorcluster)  [unwired: 1 in, 3 out]
  }
  n126 = case shown="True" w5 {
    frame False {
    }
    frame True {
      n127 = Quit LabVIEW(quit? (T)=TRUE) -> ()
    }
  }
